vi "Solve2.vi"(8 "Error In":errorcluster, 11 "object in":refnum<class "2024_10.lvclass">) -> (0 "Error Out":errorcluster, 2 "Result":u64, 3 "object out":refnum<class "2024_10.lvclass">)   [LabVIEW 2023, in "2024_10.lvclass"]
uses:
  2024_10.lvclass
  2024_10.lvclass/2024_10.ctl
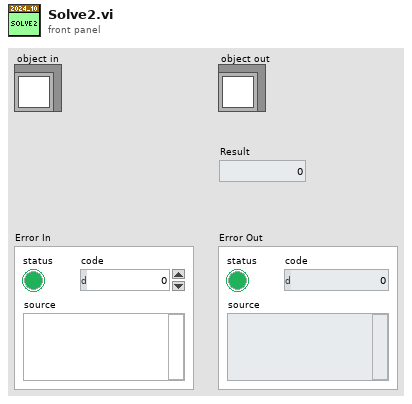
[diagram p1: front panel]
types:
  T1 = cluster{"TrailHead":cluster{i32, i32}, "TrailPeaks":cluster{i32, i32}[]}[]
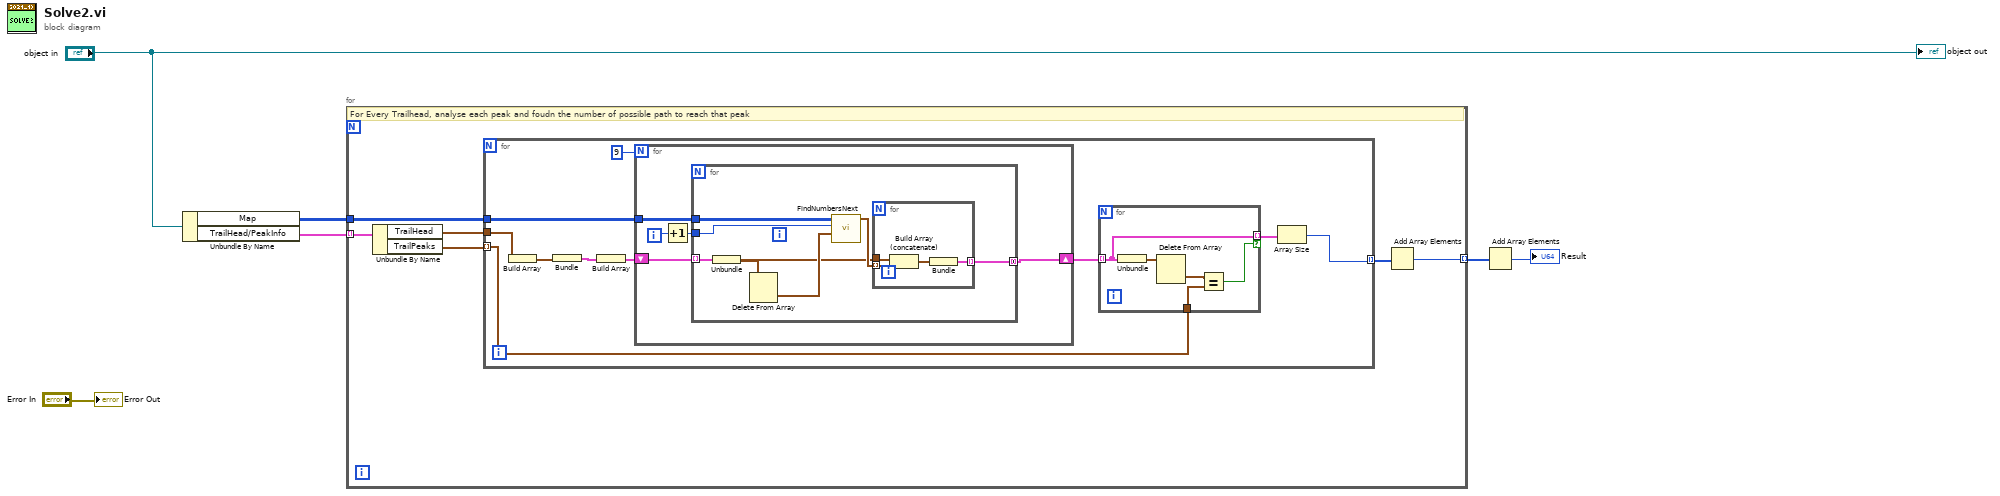
[diagram p0: block diagram]
diagram:
  n1 = Unbundle By Name("object in") -> ("Map"=w3:u8[][], "TrailHead/PeakInfo"=w4:T1)
  n2 = for {
    tunnel: w4 -> [w12] mode=indexing
    tunnel: w3 -> [w9]
    tunnel: [w7] -> w2 mode=indexing
    # "For Every Trailhead, analyse each peak and foudn the number of possible path to reach that peak"
    n3 = Unbundle By Name(w12) -> ("TrailHead"=w10:cluster{i32, i32}, "TrailPeaks"=w11:cluster{i32, i32}[])
    n4 = for {
      tunnel: w11 -> [w15] mode=indexing
      tunnel: w10 -> [w21]
      tunnel: w9 -> [w22]
      tunnel: [w13] -> w8 mode=indexing
      n5 = Build Array(w21) -> (w20:cluster{i32, i32}[])
      n6 = Bundle(w20) -> (w19:cluster{cluster{i32, i32}[]})  [unwired: 1 in]
      n7 = Build Array(w19) -> (w18:cluster{cluster{i32, i32}[]}[])
      n8 = for {
        N: 9 -> [_]
        tunnel: w22 -> [w32]
        shift-right: [w28] -> w16
        shift-left: w18 -> [w31]
        i -> [w30]
        n9 = Increment(x=w30) -> (x+1=w29:i32)
        n10 = for {
          tunnel: w32 -> [w39]
          tunnel: w31 -> [w38] mode=indexing
          tunnel: [w36] -> w28 mode=concatenating
          tunnel: w29 -> [w35]
          n11 = Unbundle(w38) -> (w33:cluster{i32, i32}[])
          n12 = Delete From Array(array=w33) -> (deleted portion=w37:cluster{i32, i32})  [unwired: 2 in, 1 out]
          n13 = call "FindNumbersNext.vi"("Cluster"=w37, "Numeric"=w35, "Map"=w39) -> ("Array"=w34:cluster{"Numeric":i32, "Numeric":i32}[])  [unwired: 8 in]
          n14 = for {
            tunnel: w33 -> [w43]
            tunnel: w34 -> [w42] mode=indexing
            tunnel: [w40] -> w36 mode=indexing
            n15 = Build Array (concatenate)(w43, w42) -> (w41:cluster{"Numeric":i32, "Numeric":i32}[])
            n16 = Bundle(w41) -> (w40:cluster{cluster{"Numeric":i32, "Numeric":i32}[]})  [unwired: 1 in]
          }
        }
      }
      n17 = for {
        tunnel: w16 -> [w23] mode=indexing
        tunnel: w15 -> [w26]
        tunnel: [w23] -> w14 mode=indexing if=w24
        n18 = Unbundle(w23) -> (w25:cluster{i32, i32}[])
        n19 = Delete From Array(array=w25) -> (deleted portion=w27:cluster{i32, i32})  [unwired: 2 in, 1 out]
        n20 = Equal?(x=w27, y=w26) -> (x = y?=w24:bool)
      }
      n21 = Array Size(array=w14) -> (size(s)=w13:i32)
    }
    n22 = Add Array Elements(numeric array=w8) -> (sum=w7:i32)
  }
  n23 = Add Array Elements(numeric array=w2) -> (sum=→"Result":i32)
  "Error Out" <- "Error In"
  "object out" <- "object in"
